vi "Database-SQLiteClose.vi"(8 "error in (no error)":errorcluster, 11 "Database-Actor in":refnum<class "Database-Actor.lvclass">) -> (0 "error out":errorcluster, 3 "Database-Actor out":refnum<class "Database-Actor.lvclass">)   [LabVIEW 2013, in "Database-Actor.lvclass"]
uses:
  Database-Actor.lvclass
  Database-Actor.lvclass/Database-Actor.ctl
  ftw-dataflow/Core/src/Database/FTW-SQLite-Connector.lvclass
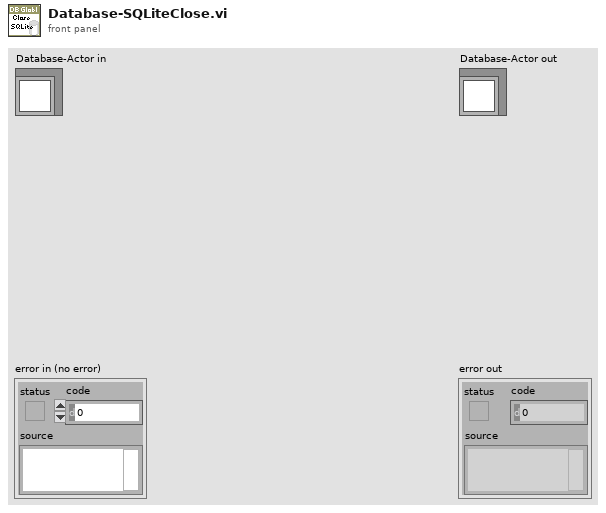
[diagram p1: front panel]
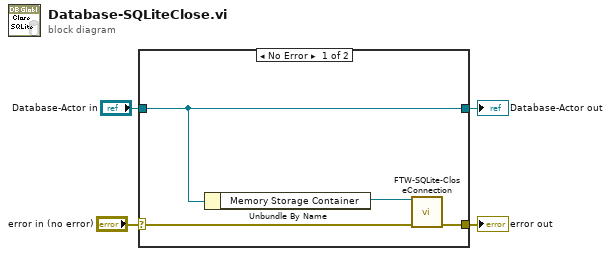
[diagram p0: block diagram]
diagram:
  n1 = case shown="No Error" "error in (no error)" {
    selector: "error in (no error)" -> [w6 w10]
    tunnel: [w5 w10] -> w3
    tunnel: [w8 w9] -> w1
    tunnel: "Database-Actor in" -> [w8 w9]
    frame No Error {
      n2 = Unbundle By Name(w8) -> ("Memory Storage Container"=w7:refnum<class "FTW-SQLite-Connector.lvclass">)
      n3 = call "FTW-SQLite-CloseConnection.vi"("SQLite Connector"=w7, "error in"=w6) -> ("error out"=w5:errorcluster)  [unwired: 13 in]
    }
    frame Error {
    }
  }
  "error out" <- w3
  "Database-Actor out" <- w1
